vi "DelayGenerator-StaticBaseline.vi"(2 "site_info":T4 {"longitude" format="%_10g"; "latitude" format="%_10g"}, 3 "Time Stamp":timestamp, 5 "Baseline":T3 {"Up" format="%.6g"; "North" format="%.6g"; "East" format="%.6g"}, 7 "dt":dbl[unit]=66.131, 8 "cat_entry":T2 {"dec" format="%.6g"; "ra" format="%.6g"}, 9 "error in (no error)":errorcluster caption="error out") -> (6 "error out":errorcluster)   [LabVIEW 2009]
uses:
  Controls/SiteInformation.ctl
  Controls/Baseline.ctl
  Controls/StarAstrometricEntry.ctl
  Controls/DelayTarget.ctl
  <vilib>/Analysis/baseanly.llb/Real Dot Product.vi
  <vilib>/Analysis/NI_AALBase.lvlib
panel:
  out "DelayTarget":T1
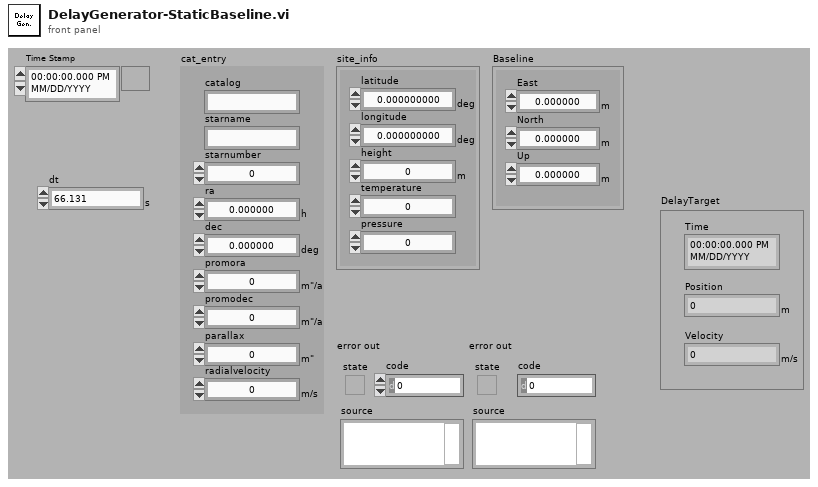
[diagram p1: front panel]
types:
  T1 = typedef "DelayTarget.ctl" = cluster{"Time":timestamp, "Position":dbl[unit], "Velocity":dbl[unit]}
  T2 = typedef "StarAstrometricEntry.ctl" = cluster{"catalog":string, "starname":string, "starnumber":i32, "ra":dbl[unit], "dec":dbl[unit], "promora":dbl[unit], "promodec":dbl[unit], "parallax":dbl[unit], "radialvelocity":dbl[unit]}
  T3 = typedef "Baseline.ctl" = cluster{"East":dbl[unit], "North":dbl[unit], "Up":dbl[unit]}
  T4 = typedef "SiteInformation.ctl" = cluster{"latitude":dbl[unit], "longitude":dbl[unit], "height":dbl[unit], "temperature":dbl, "pressure":dbl}
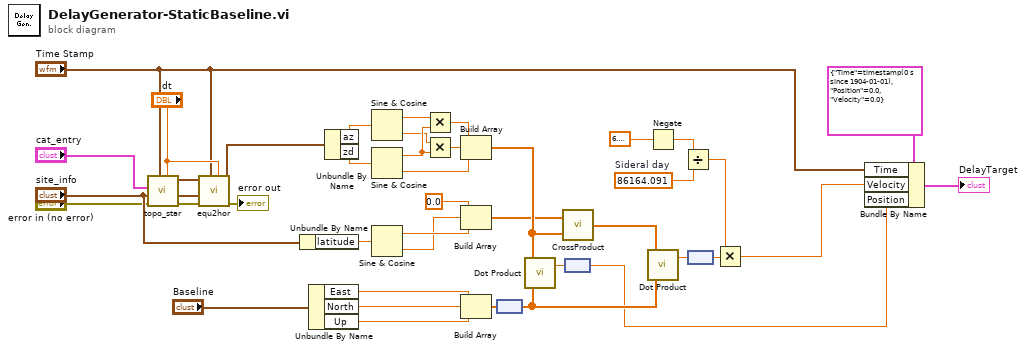
[diagram p0: block diagram]
diagram:
  w10 = dbl[unit] 86164.091  # Sideral day
  n1 = call "topo_star.vi"("deltat (TT-UT1)"="dt", "TimeStamp [UT1]"="Time Stamp", "error in (no error)"="error in (no error)", "on_surface"="site_info", "cat_entry"="cat_entry") -> ("error out"=w15:errorcluster, "ra/dec"=w16:cluster{"ra":dbl[unit], "dec":dbl[unit]})  [unwired: 3 in]
  n2 = call "equ2hor.vi"("deltat [TT-UT1]"="dt", "TimeStamp [UT1]"="Time Stamp", "error in (no error)"=w15, "on_surface"="site_info", "ra/dec"=w16) -> ("error out"=→"error out":errorcluster, "az/zd"=w14:cluster{"az":dbl[unit], "zd":dbl[unit]})  [unwired: 2 in, 1 out]
  n3 = Unbundle By Name("site_info") -> ("latitude"=w36:dbl[unit])
  n4 = Unbundle By Name("Baseline") -> ("East"=w23:dbl[unit], "North"=w22:dbl[unit], "Up"=w24:dbl[unit])
  n5 = Unbundle By Name(w14) -> ("az"=w33:dbl[unit], "zd"=w26:dbl[unit])
  n6 = Sine & Cosine(0:w33) -> (1:w28:dbl, 2:w27:dbl)
  n7 = Sine & Cosine(0:w26) -> (1:w29:dbl, 2:w32:dbl)
  n8 = Sine & Cosine(0:w36) -> (1:w13:dbl, 2:w12:dbl)
  n9 = Multiply(x=w28, y=w29) -> (x*y=w30:dbl)
  n10 = Multiply(x=w27, y=w29) -> (x*y=w31:dbl)
  n11 = Build Array(w30, w31, w32) -> (w11:dbl[])
  n12 = Build Array(0.0 ("élément"), w12, w13) -> (w8:dbl[])
  n13 = Build Array(w23, w22, w24) -> (w21:dbl[unit][])
  n14 = node(w21) -> (w40:dbl[])
  n15 = call-poly <vilib>:"Dot Product.vi"("Y Vector"=w40, "X Vector"=w11) -> ("X * Y"=w25:dbl)  [unwired: 1 out]
  n16 = call "CrossProduct.vi"("V2"=w11, "V1"=w8) -> ("V1^V2"=w39:dbl[])
  n17 = node(w25) -> (w3:dbl[unit])
  n18 = Negate(x=6.283185307179586) -> (-x=w6:dbl)
  n19 = call-poly <vilib>:"Dot Product.vi"("Y Vector"=w40, "X Vector"=w39) -> ("X * Y"=w38:dbl)  [unwired: 1 out]
  n20 = Divide(x=w6, y=w10) -> (x/y=w9:dbl[unit])
  n21 = node(w38) -> (w41:dbl[unit])
  n22 = Multiply(x=w9, y=w41) -> (x*y=w2:dbl[unit])
  n23 = Bundle By Name(cluster=T1 {"Time"=timestamp(0 s since 1904-01-01), "Position"=0.0, "Velocity"=0.0} ("DelayTarget"), "Time"="Time Stamp", "Velocity"=w2, "Position"=w3) -> (→"DelayTarget":T1)
